vi "configuration UI.vi"() -> ()   [LabVIEW 2013, in "TDMS datalogger editor node.lvclass"]
uses:
  TDMS datalogger editor node.lvclass
  <vilib>/CEF_TreeControl/Node/NodeRef.ctl
  <vilib>/CEF_TreeControl/Node/NISE_CEF_Node.lvclass
  <vilib>/NI/AMC/Message Queue.ctl
  <vilib>/NI/AMC/Message.ctl
  <vilib>/NI/Tools/Keyed Array/KeyedArray.ctl
  <vilib>/CEF_TreeControl/Node/UserEventRef.ctl
  <vilib>/CEF_TreeControl/Controls/EventCluster.ctl
  <vilib>/NI/TBM Modules/TDMS Datalogger/module/configuration/TDMS datalogger configuration.lvclass
  <vilib>/NI/Tag Bus Data Framework/Configuration Editor/Classes/Engine Parent/Engine Parent Editor Node.lvclass
  <vilib>/NI/Tag Bus/tag/tag descriptor.lvclass
  <vilib>/NI/Tag Bus/tag/Data Type.ctl
  <vilib>/NI/Module Execution Interface/Engine Configuration/engine configuration.lvclass
  <vilib>/NI/Tag Bus/tag/tag descriptor.lvclass/tag descriptor.ctl
  <vilib>/NI/Tag Bus Module Framework/root configuration/TBM configuration.lvclass/TBM configuration.ctl
  <vilib>/NI/TBM Modules/TDMS Datalogger/module/configuration/TDMS datalogger configuration.lvclass/TDMS datalogger configuration.ctl
  TDMS datalogger editor node.lvclass/TDMS datalogger editor node.ctl
  <vilib>/NI/Tag Bus/tag/write tag name.vi
  <vilib>/NI/Tag Bus/tag/write data type.vi
  <vilib>/NI/TBM Modules/TDMS Datalogger/module/configuration/Write scans per write.vi
  <vilib>/NI/TBM Modules/TDMS Datalogger/module/configuration/Write queue size.vi
  <vilib>/NI/TBM Modules/TDMS Datalogger/module/configuration/Write Path.vi
  <vilib>/NI/TBM Modules/TDMS Datalogger/module/configuration/Write backup directory.vi
  <vilib>/NI/TBM Modules/TDMS Datalogger/module/configuration/Write channel pattern matches.vi
  <vilib>/NI/Tag Bus Module Framework/root configuration/Read instance name.vi
  <vilib>/NI/TBM Modules/TDMS Datalogger/module/configuration/Read backup directory.vi
  <vilib>/NI/TBM Modules/TDMS Datalogger/module/configuration/Read Path.vi
  <vilib>/NI/TBM Modules/TDMS Datalogger/module/configuration/Read queue size.vi
  <vilib>/NI/TBM Modules/TDMS Datalogger/module/configuration/Read scans per write.vi
  <vilib>/NI/TBM Modules/TDMS Datalogger/module/configuration/Read add enable channel.vi
  <vilib>/NI/TBM Modules/TDMS Datalogger/module/configuration/Read channel pattern matches.vi
  <vilib>/NI/Tag Bus Data Framework/Configuration Editor/Classes/Module editor node/Read Module Configuration.vi
  <vilib>/NI/Tag Bus Module Framework/root configuration/create GUID.vi
  <vilib>/NI/Tag Bus Module Framework/module configuration/TBM module configuration.lvclass
  <vilib>/NI/Tag Bus Data Framework/Configuration Editor/Classes/Module editor node/module editor node.lvclass
  <vilib>/CEF_TreeControl/NISE_CEF_TreeControl.lvlib
  <vilib>/NI/Tools/Keyed Array/Tools_KeyedArray.lvlib
  <vilib>/NI/AMC/AMC.lvlib
panel:
  in  "Tab Control":T1(tab)
  in  "channels":i32(listbox)
  in  "remove":bool
  in  "avail tags":i32(listbox)=-1
  in  "add all":bool
  in  "add1":bool
  out "Enable Tag":string
  in  "history error":bool
  in  "path error":bool
  in  "Historical Directory":path
  in  "use enable channel":bool
  in  "recalc":bool
  out "Approximate memory usage":dbl
  in  "queue size":i32=2
  in  "scans per write":i32=20
  in  "File Path":path
  in  "Channel Subscription Pattern Matches":string[](array[string])
  in  "Enable Dynamic Mapping":bool
  in  "user event":T2
  in  "main queue":T3
  in  "node ref":T4
  # "kB"
  # "Note: This value ignores dynamic mapping"
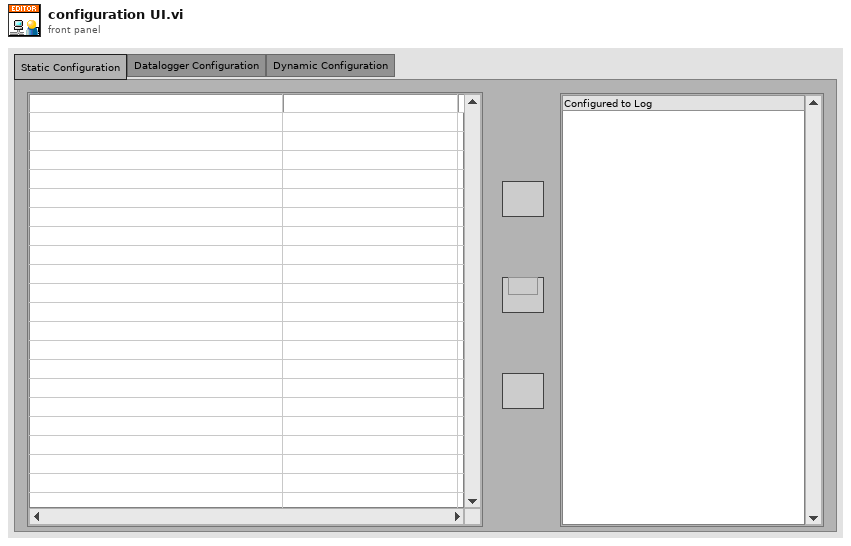
[diagram p1: front panel]
types:
  T1 = enum32{"Static Configuration", "Datalogger Configuration", "Dynamic Configuration"}
  T2 = typedef "NISE_CEF_Node.lvclass/UserEventRef.ctl" = refnum<user-event>
  T3 = typedef "AMC.lvlib/Message Queue.ctl" = refnum<queue>
  T4 = typedef "NISE_CEF_Node.lvclass/NodeRef.ctl" = refnum<data-value>
  T5 = typedef "NISE_CEF_TreeControl.lvlib/EventCluster.ctl" = cluster{"command":string, "data":string}
  T6 = typedef "tag bus.lvlib/tag descriptor.lvclass/Data Type.ctl" = enum16{"Double", "Single", "I64", "I32", "I16", "I8", "U64", "U32", "U16", "U8", "Boolean", "String", "Array of Double", "Array of Single", "Array of I64", "Array of I32", "Array of I16", "Array of I8", "Array of U64", "Array of U32", "Array of U16", "Array of U8", "Array of Boolean", "Array of String"}
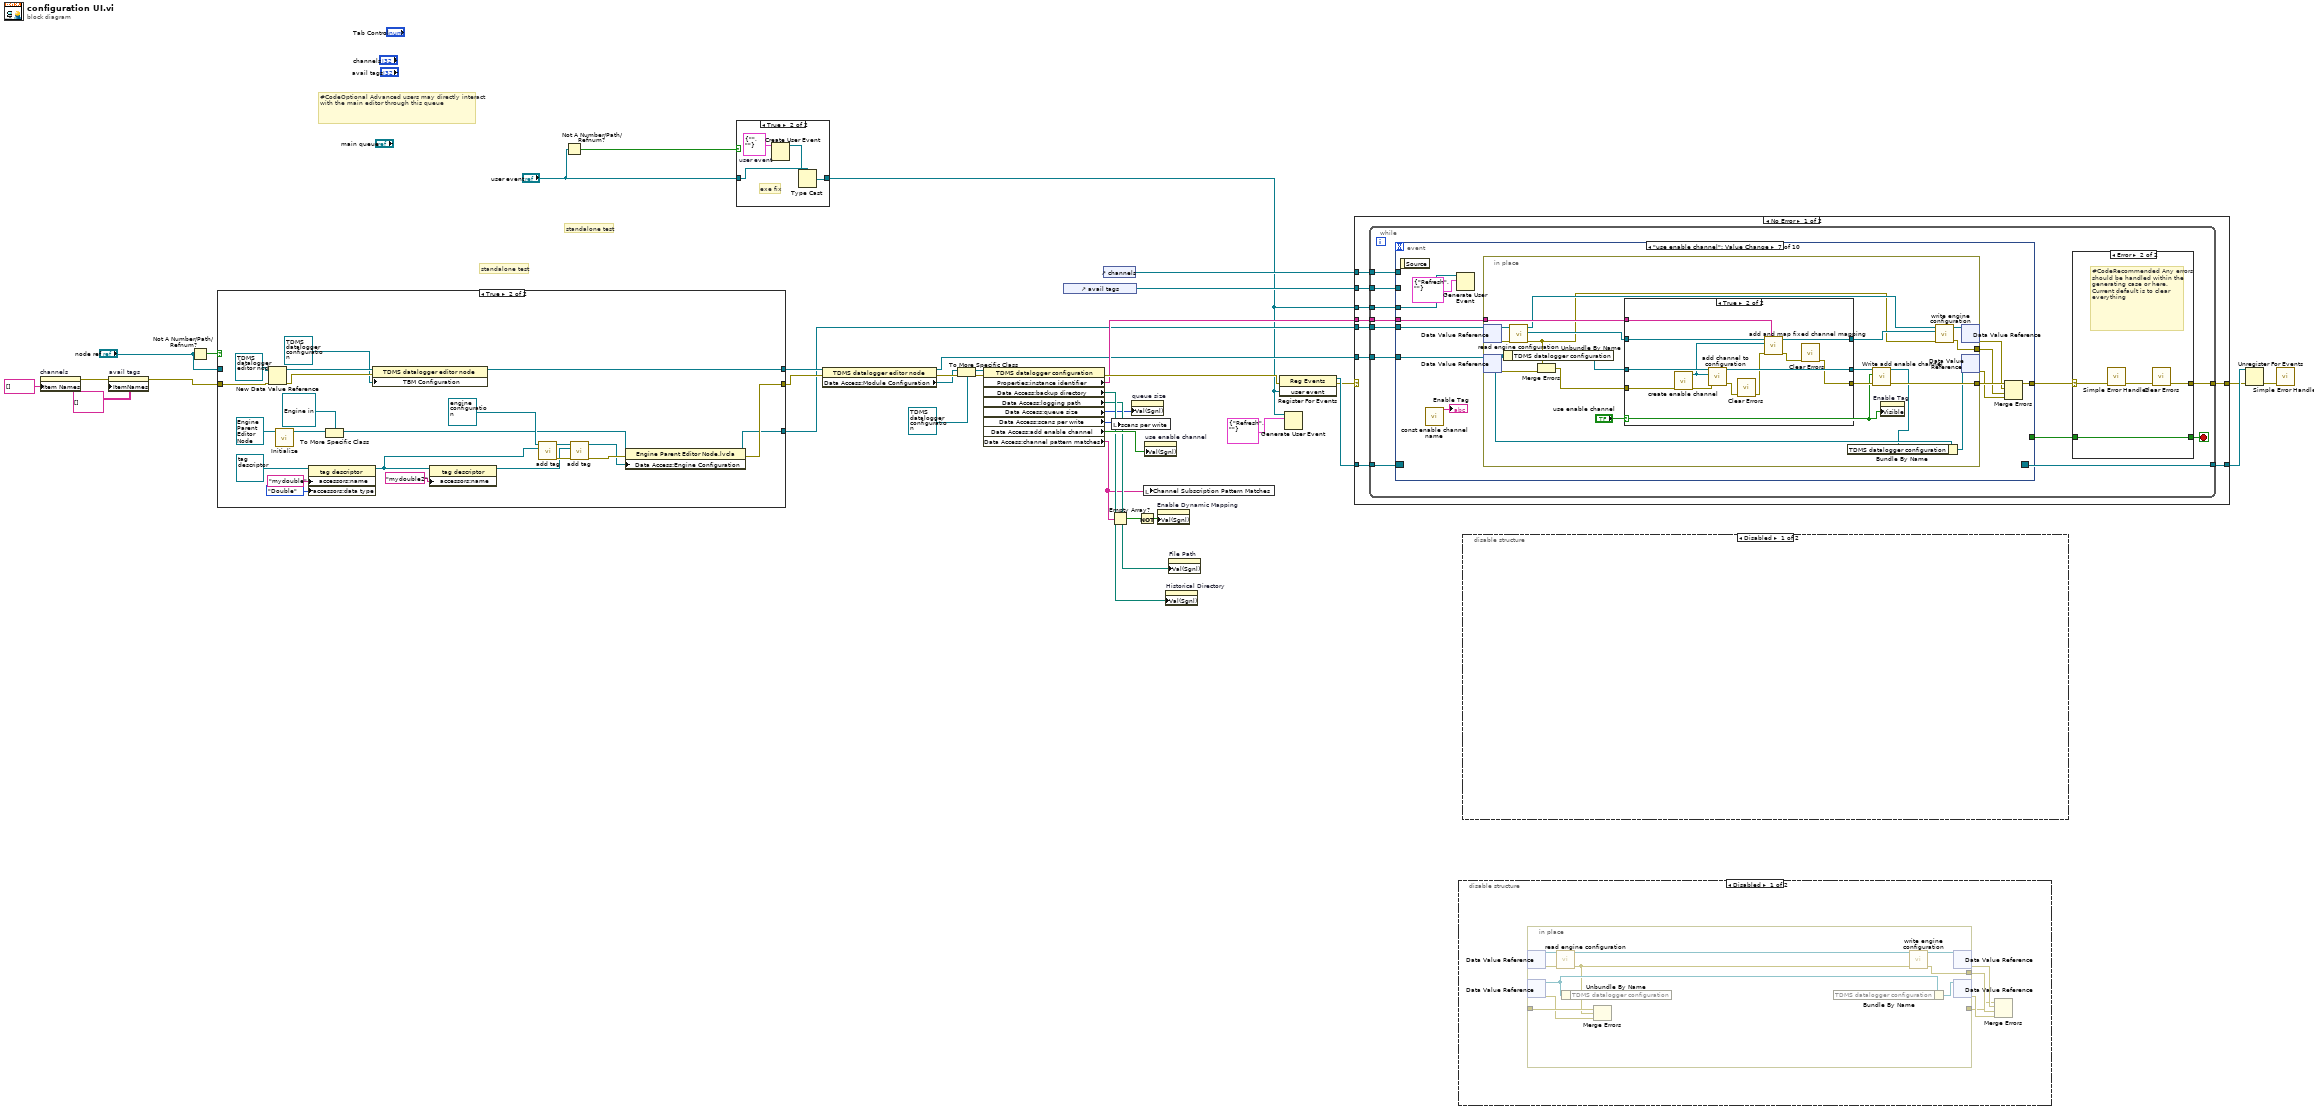
[diagram p0: block diagram]
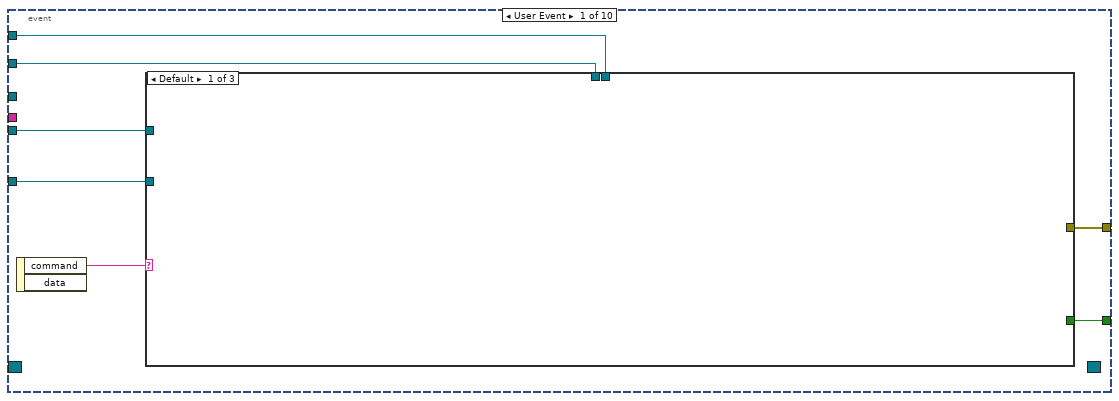
[diagram p4: hidden frame]
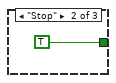
[diagram p5: hidden frame]
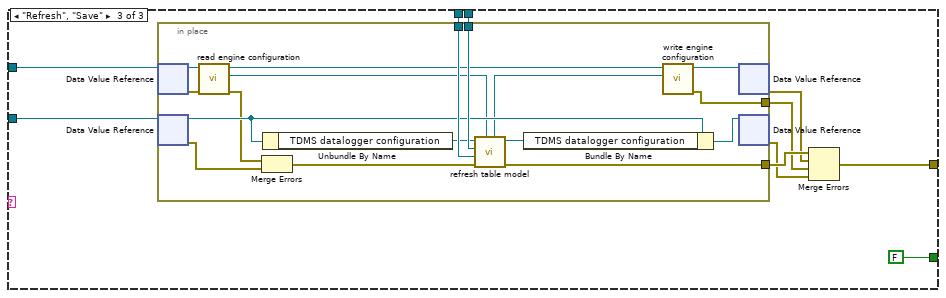
[diagram p6: hidden frame]
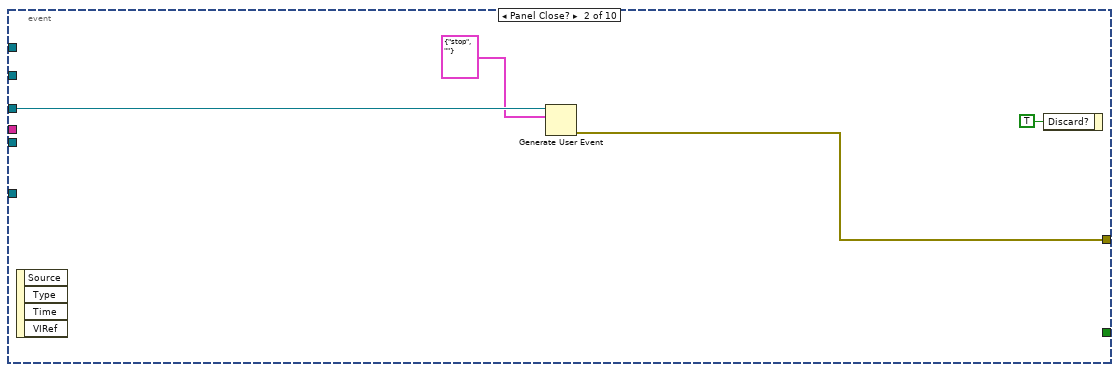
[diagram p7: hidden frame]
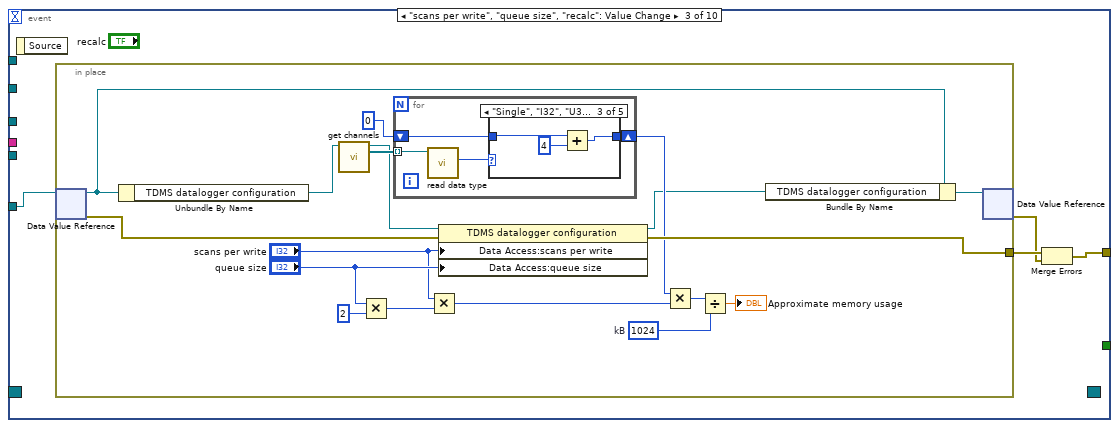
[diagram p8: hidden frame]
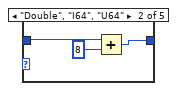
[diagram p10: hidden frame]
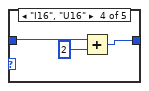
[diagram p11: hidden frame]
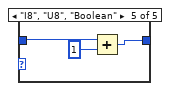
[diagram p12: hidden frame]
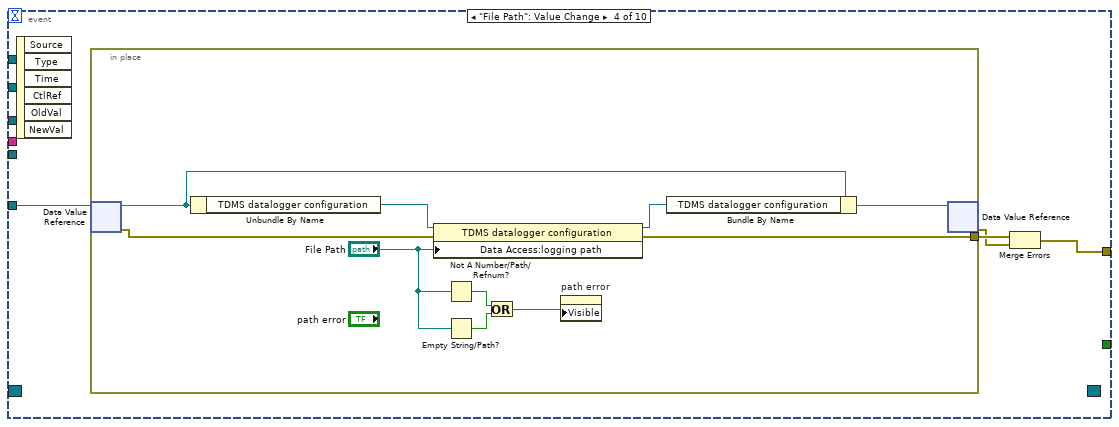
[diagram p13: hidden frame]
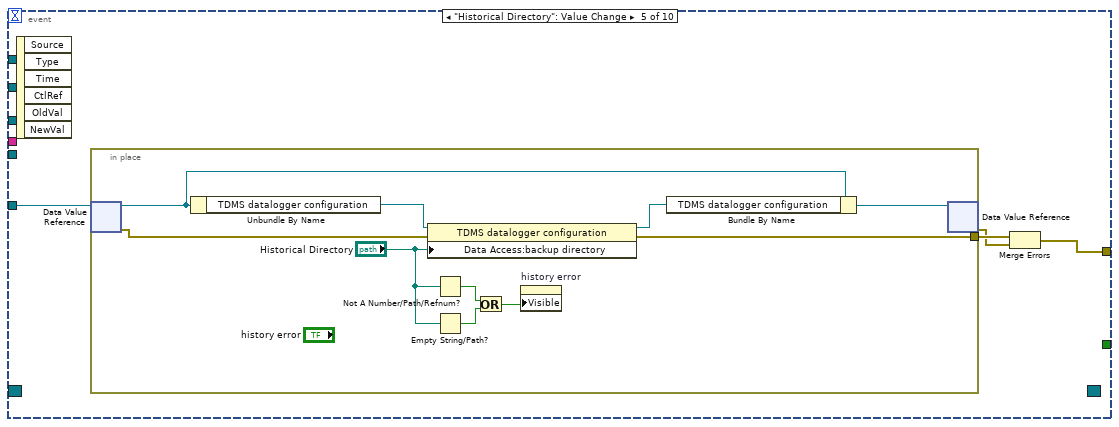
[diagram p14: hidden frame]
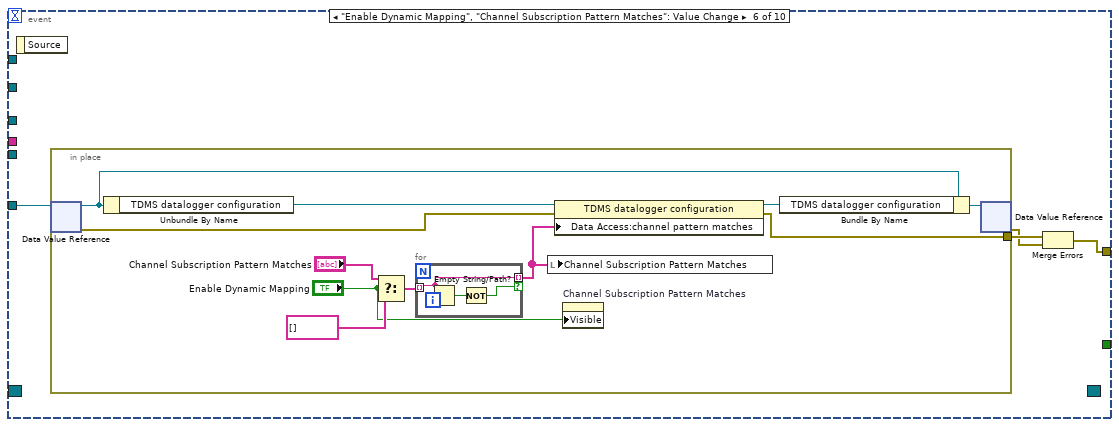
[diagram p15: hidden frame]
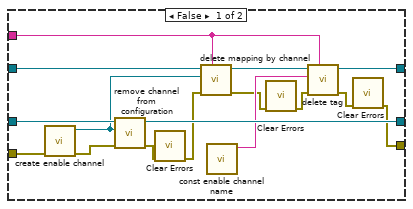
[diagram p16: hidden frame]
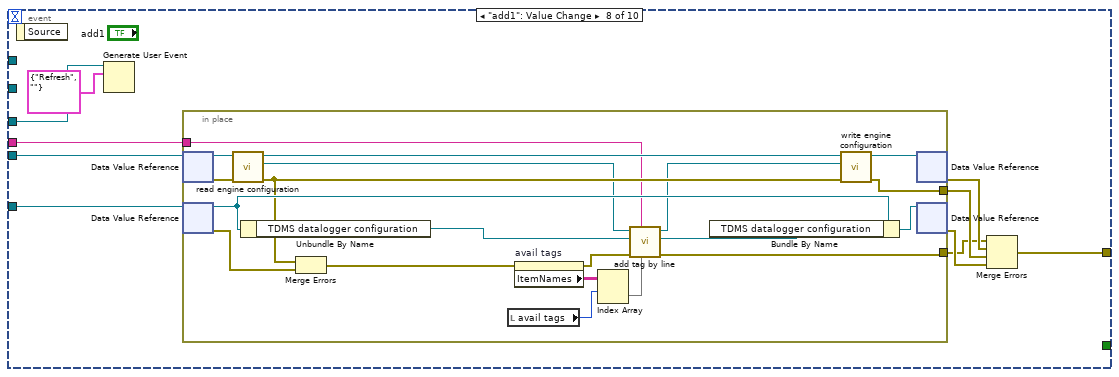
[diagram p17: hidden frame]
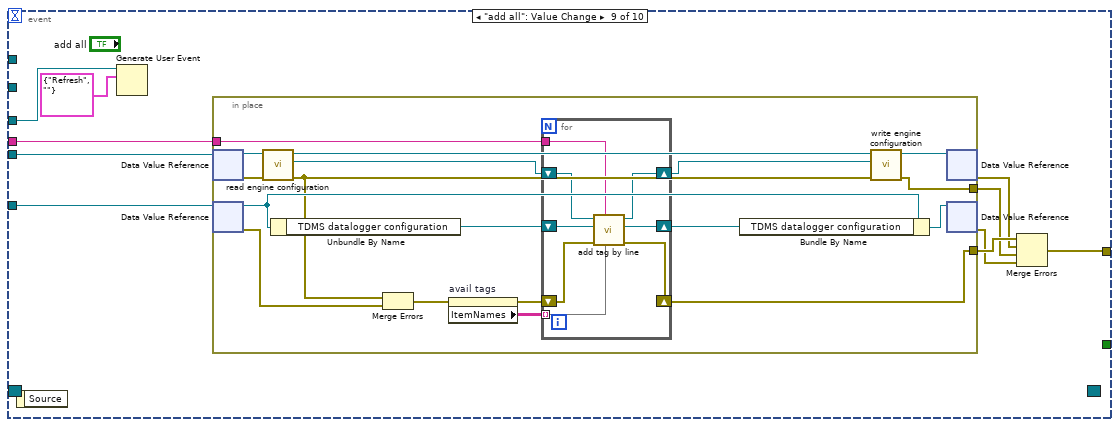
[diagram p18: hidden frame]
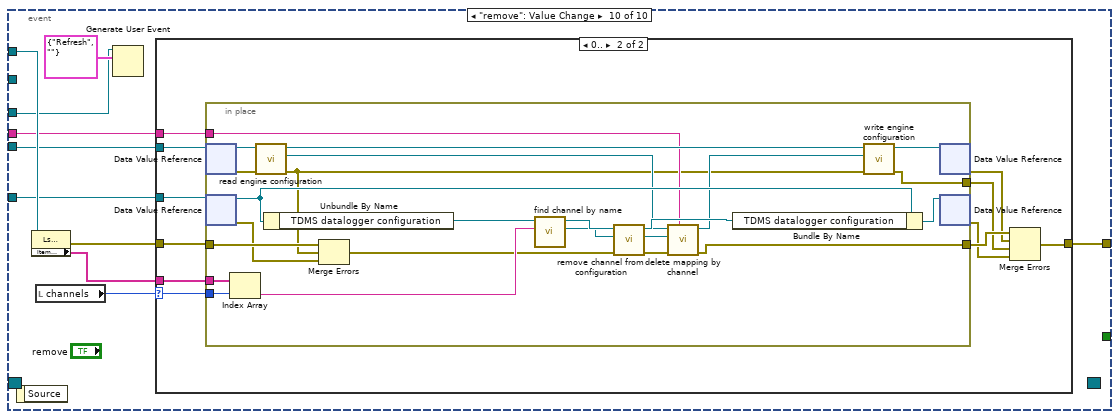
[diagram p19: hidden frame]
diagram:
  # "standalone test"
  # "standalone test"
  # "#CodeOptional Advanced users may directly interact with the main editor through this queue"
  n1 = property on="channels" class="LstBox (strict)"("Item Names"=string[] []) -> (error out=w16:errorcluster)  [unwired: 2 in, 1 out]
  n2 = property on="avail tags" class="MCListbox (strict)"(error in=w16, "ItemNames"=string[][] [] ("Item Names")) -> (error out=w5:errorcluster)  [unwired: 1 in, 1 out]
  n3 = Not A Number/Path/Refnum?(number/path/refnum="node ref") -> (NaN/Path/Refnum?=w7:bool)
  n4 = case shown="True" w7 {
    tunnel: "node ref" -> [w42 _]
    tunnel: [w41 w66] -> w9
    tunnel: [w40 w47] -> w8
    tunnel: [w39 w45] -> w4
    tunnel: w5 -> [w37 w49]
    frame False {
      n5 = call <vilib>:"locate engine.vi"("error in"=w37, "component"=w42) -> ("error out"=w38:errorcluster, "engine"=w39:refnum<data-value>)  [unwired: 8 in]
      n6 = To More Specific Class(target class=refnum<data-value> refnum ("data value reference"), reference=w42, error in=w38) -> (specific class reference=w41:refnum<data-value>, error out=w40:errorcluster)
    }
    frame True {
      n7 = New Data Value Reference(data value=refnum<class "TDMS datalogger editor node.lvclass"> refnum ("tag bus configurable plugin editor node"), error in=w49) -> (data value reference=w65:refnum<data-value>, error out=w50:errorcluster)
      n8 = call-dynamic "Initialize.vi"("Engine in"=refnum<class "Engine Parent Editor Node.lvclass"> refnum) -> ("data value reference"=w64:T4)  [unwired: 8 in, 2 out]
      n9 = property class="tag descriptor"(reference=refnum<class "tag descriptor.lvclass"> refnum ("tag descriptor"), "accessors:name"="mydouble" ("name"), "accessors:data type"=Data_Type."Double" ("data type")) -> (reference out=w53:refnum<class "tag descriptor.lvclass">)  [unwired: 1 in, 1 out]
      n10 = To More Specific Class(target class=refnum<data-value> refnum ("data value reference"), reference=w64) -> (specific class reference=w46:refnum<data-value>)  [unwired: 1 in, 1 out]
      n11 = property class="TDMS datalogger editor node"(reference=w65, error in=w50, "TBM Configuration"=refnum<class "TDMS datalogger configuration.lvclass"> refnum ("TDMS datalogger configuration")) -> (reference out=w66:refnum<data-value>)  [unwired: 1 out]
      n12 = property class="tag descriptor"(reference=w53, "accessors:name"="mydouble2" ("name")) -> (reference out=w54:refnum<class "tag descriptor.lvclass">)  [unwired: 1 in, 1 out]
      n13 = call <vilib>:"add tag.vi"("tag descriptor"=w53, "engine configuration in"=refnum<class "engine configuration.lvclass"> refnum ("Engine Configuration")) -> ("error out"=w57:errorcluster, "engine configuration out"=w56:refnum<class "engine configuration.lvclass">)  [unwired: 8 in]
      n14 = call <vilib>:"add tag.vi"("error in"=w57, "tag descriptor"=w54, "engine configuration in"=w56) -> ("error out"=w55:errorcluster, "engine configuration out"=w44:refnum<class "engine configuration.lvclass">)  [unwired: 7 in]
      n15 = property class="Engine Parent Editor Node.lvcla"(reference=w46, error in=w55, "Data Access:Engine Configuration"=w44) -> (reference out=w45:refnum<data-value>, error out=w47:errorcluster)
    }
  }
  n16 = Not A Number/Path/Refnum?(number/path/refnum="user event") -> (NaN/Path/Refnum?=w11:bool)
  n17 = case shown="True" w11 {
    tunnel: [w67 w70] -> w3
    tunnel: "user event" -> [w67 w71]
    frame False {
    }
    frame True {
      w68 = T5 {"command"="", "data"=""}  # user event
      # "exe fix"
      n18 = Create User Event(user event datatype=w68) -> (user event=w69:refnum<user-event>)  [unwired: 1 in, 1 out]
      n19 = Type Cast(type=w71, x=w69) -> (*(type *) &x=w70:T2)
    }
  }
  n20 = property class="TDMS datalogger editor node"(reference=w9, error in=w8) -> (reference out=w12:refnum<data-value>, error out=w33:errorcluster, "Data Access:Module Configuration"=w23:refnum<class "TBM module configuration.lvclass">)
  n21 = To More Specific Class(target class=refnum<class "TDMS datalogger configuration.lvclass"> refnum ("TDMS datalogger configuration"), reference=w23, error in=w33) -> (specific class reference=w21:refnum<class "TDMS datalogger configuration.lvclass">, error out=w24:errorcluster)
  n22 = property class="TDMS datalogger configuration"(reference=w21, error in=w24) -> (error out=w20:errorcluster, "Properties:instance identifier"=w17:string, "Data Access:backup directory"=w30:path, "Data Access:logging path"=w29:path, "Data Access:queue size"=w28:i32, "Data Access:scans per write"=w32:i32, "Data Access:add enable channel"=w31:bool, "Data Access:channel pattern matches"=w27:string[])  [unwired: 1 out]
  n23 = control-ref of="avail tags"() -> (w18:refnum<vi>)
  n24 = control-ref of="channels"() -> (w19:refnum<vi>)
  n25 = Empty Array?(array=w27) -> (empty?=w25:bool)
  n26 = local write "scans per write"(w32) -> ()
  n27 = property on="queue size" class="DigNum (strict)"("Val(Sgnl)"=w28) -> ()  [unwired: 2 in, 2 out]
  n28 = Not(x=w25) -> (.not. x?=w26:bool)
  n29 = local write "Channel Subscription Pattern Matches"(w27) -> ()
  n30 = property on="use enable channel" class="Bool (strict)"("Val(Sgnl)"=w31) -> ()  [unwired: 2 in, 2 out]
  n31 = property on="Enable Dynamic Mapping" class="Bool (strict)"("Val(Sgnl)"=w26) -> ()  [unwired: 2 in, 2 out]
  n32 = property on="Historical Directory" class="Path"("Val(Sgnl)"=w30) -> ()  [unwired: 2 in, 2 out]
  n33 = property on="File Path" class="Path"("Val(Sgnl)"=w29) -> ()  [unwired: 2 in, 2 out]
  n34 = register-events(error in=w20, w3) -> (reference out=w36:refnum<event-registration>, error out=w1:errorcluster)  [unwired: 1 in]
  n35 = Generate User Event(user event=w3, event data cluster=T5 {"command"="Refresh", "data"=""} ("event data")) -> ()  [unwired: 2 in, 2 out]
  n36 = case shown="No Error" w1 {
    selector: w1 -> [_ w393]
    tunnel: w36 -> [w80 w392]
    tunnel: [w79 w392] -> w35
    tunnel: w19 -> [w78 _]
    tunnel: w18 -> [w77 _]
    tunnel: w17 -> [w76 _]
    tunnel: [w75 w393] -> w13
    tunnel: w12 -> [w74 _]
    tunnel: w4 -> [w73 _]
    tunnel: w3 -> [w72 _]
    frame No Error {
      n37 = while {
        tunnel: w80 -> [w92]
        tunnel: [w91] -> w79
        tunnel: w78 -> [w87]
        tunnel: w77 -> [w86]
        tunnel: w76 -> [w81]
        tunnel: w73 -> [w85]
        tunnel: w74 -> [w84]
        tunnel: w72 -> [w83]
        tunnel: [w88] -> w75
        stop <- w89 stop-if-true
        n38 = event shown="[6] \"use enable channel\": Value Change" {
          selector: w92 -> [_ _ _ _ _ _ _ _ _ _]
          dyn-events: [_ _ _ _ _ _ _ _ _ _] -> w91
          timeout: _ -> [_ _ _ _ _ _ _ _ _ _]
          tunnel: [w105 _ _ _ _ _ _ _ _ _] -> w82
          tunnel: [w103 w136 w139 w179 w193 w205 w229 w282 w314 w356] -> w90
          tunnel: w87 -> [w100 _ _ _ _ _ _ _ _ w354]
          tunnel: w86 -> [w99 _ _ _ _ _ _ _ _ _]
          tunnel: w85 -> [w102 _ _ _ _ _ w227 w283 w312 w347]
          tunnel: w84 -> [w101 _ w140 w178 w192 w206 w228 w284 w313 w348]
          tunnel: w83 -> [_ w135 _ _ _ _ w231 w289 w319 w349]
          tunnel: w81 -> [_ _ _ _ _ _ w233 w281 w311 w352]
          event User Event {
            n39 = event-data() -> ("command"=w104:string)  [unwired: 1 in, 1 out]
            n40 = case shown="Default" w104 {
              tunnel: [_ TRUE FALSE] -> w105
              tunnel: [_ _ w112] -> w103
              tunnel: w102 -> [_ _ w111]
              tunnel: w101 -> [_ _ w110]
              tunnel: w100 -> [_ _ w114]
              tunnel: w99 -> [_ _ w113]
              frame Default {
              }
              frame "Stop" {
              }
              frame "Refresh", "Save" {
                n41 = in-place {
                  in-place-border: [w133] -> w115
                  in-place-border: w114 -> [w132]
                  in-place-border: w113 -> [w131]
                  in-place-border: [w117] -> w109
                  n42 = in-place-dvr #1(w111) -> (w121:refnum<class "Engine Parent Editor Node.lvclass">, w122:errorcluster)
                  n43 = in-place-dvr #2(w110) -> (w128:refnum<class "TDMS datalogger editor node.lvclass">, w125:errorcluster)
                  n44 = call <vilib>:"read engine configuration.vi"("error in"=w122, "Engine Parent Editor Node in"=w121) -> ("error out"=w118:errorcluster, "engine configuration"=w119:refnum<class "engine configuration.lvclass">, "Engine Parent Editor Node out"=w120:refnum<class "Engine Parent Editor Node.lvclass">)  [unwired: 7 in]
                  n45 = Merge Errors(w118, w125) -> (w130:errorcluster)
                  n46 = Unbundle By Name(w128) -> ("TDMS datalogger configuration"=w129:refnum<class "TDMS datalogger configuration.lvclass">)
                  n47 = call "refresh table model.vi"("engine configuration"=w119, "error in"=w130, "avail tags"=w131, "chan table"=w132, "TDMS datalogger configuration"=w129) -> ("error out"=w133:errorcluster, "TDMS datalogger configuration out"=w126:refnum<class "TDMS datalogger configuration.lvclass">, "engine configuration out"=w123:refnum<class "engine configuration.lvclass">)  [unwired: 4 in]
                  n48 = Bundle By Name(cluster=w128, "TDMS datalogger configuration"=w126) -> (w127:refnum<class "TDMS datalogger editor node.lvclass">)
                  n49 = call <vilib>:"write engine configuration.vi"("engine configuration"=w123, "Engine Parent Editor Node in"=w120) -> ("error out"=w117:errorcluster, "Engine Parent Editor Node out"=w124:refnum<class "Engine Parent Editor Node.lvclass">)  [unwired: 8 in]
                  n50 = in-place-dvr #1(w124) -> (w108:errorcluster)  [unwired: 1 out]
                  n51 = in-place-dvr #2(w127) -> (w107:errorcluster)  [unwired: 1 out]
                }
                n52 = Merge Errors(w115, w108, w109, w107) -> (w112:errorcluster)
              }
            }
          }
          event Panel Close? {
            n53 = event-data() -> ()  [unwired: 1 in, 4 out]
            n54 = Generate User Event(user event=w135, event data cluster=T5 {"command"="stop", "data"=""} ("event data")) -> (error out=w136:errorcluster)  [unwired: 2 in, 1 out]
            n55 = event-data("Discard?"=TRUE) -> ()  [unwired: 1 in, 1 out]
          }
          event "scans per write", "queue size", "recalc": Value Change {
            n56 = event-data() -> ()  [unwired: 1 in, 1 out]
            n57 = in-place {
              in-place-border: [w159] -> w141
              w153 = u32 1024  # kB
              n58 = in-place-dvr #3(w140) -> (w145:refnum<class "TDMS datalogger editor node.lvclass">, w146:errorcluster)
              n59 = Unbundle By Name(w145) -> ("TDMS datalogger configuration"=w143:refnum<class "TDMS datalogger configuration.lvclass">)
              n60 = call-dynamic "get channels.vi"("module configuration in"=w143) -> ("channels"=w149:refnum<class "TBM channel.lvclass">[], "module configuration out"=w147:refnum<class "TDMS datalogger configuration.lvclass">)  [unwired: 9 in]
              n61 = Multiply(x="queue size", y=2 ("x")) -> (x*y=w158:i32)
              n62 = for {
                shift-right: [w162] -> w150
                shift-left: u32 0 -> [w163]
                tunnel: w149 -> [w160] mode=indexing
                n63 = call <vilib>:"read data type.vi"("system tag in"=w160) -> ("data type"=w161:T6)  [unwired: 8 in, 2 out]
                n64 = case shown="\"Single\", \"I32\", \"U32\"" w161 {
                  tunnel: w163 -> [w164 w167 w170 w173 w176]
                  tunnel: [w164 w166 w169 w172 w175] -> w162
                  frame Default {
                  }
                  frame "Double", "I64", "U64" {
                    n65 = Add(x=w167, y=u32 8) -> (x+y=w166:u32)
                  }
                  frame "Single", "I32", "U32" {
                    n66 = Add(x=w170, y=u32 4) -> (x+y=w169:u32)
                  }
                  frame "I16", "U16" {
                    n67 = Add(x=w173, y=u32 2) -> (x+y=w172:u32)
                  }
                  frame "I8", "U8", "Boolean" {
                    n68 = Add(x=w176, y=u32 1) -> (x+y=w175:u32)
                  }
                }
              }
              n69 = Multiply(x="scans per write", y=w158) -> (x*y=w152:i32)
              n70 = property class="TDMS datalogger configuration"(reference=w147, error in=w146, "Data Access:scans per write"="scans per write", "Data Access:queue size"="queue size") -> (reference out=w142:refnum<class "TDMS datalogger configuration.lvclass">, error out=w159:errorcluster)
              n71 = Multiply(x=w150, y=w152) -> (x*y=w154:u32)
              n72 = Divide(x=w154, y=w153) -> (x/y=→"Approximate memory usage":dbl)
              n73 = Bundle By Name(cluster=w145, "TDMS datalogger configuration"=w142) -> (w144:refnum<class "TDMS datalogger editor node.lvclass">)
              n74 = in-place-dvr #3(w144) -> (w138:errorcluster)  [unwired: 1 out]
            }
            n75 = Merge Errors(w141, w138) -> (w139:errorcluster)
          }
          event "File Path": Value Change {
            n76 = event-data() -> ()  [unwired: 1 in, 6 out]
            n77 = in-place {
              in-place-border: [w190] -> w180
              n78 = in-place-dvr #4(w178) -> (w181:refnum<class "TDMS datalogger editor node.lvclass">, w184:errorcluster)
              n79 = Unbundle By Name(w181) -> ("TDMS datalogger configuration"=w185:refnum<class "TDMS datalogger configuration.lvclass">)
              n80 = property class="TDMS datalogger configuration"(reference=w185, error in=w184, "Data Access:logging path"="File Path") -> (reference out=w183:refnum<class "TDMS datalogger configuration.lvclass">, error out=w190:errorcluster)
              n81 = Not A Number/Path/Refnum?(number/path/refnum="File Path") -> (NaN/Path/Refnum?=w187:bool)
              n82 = Empty String/Path?(string/path="File Path") -> (empty?=w188:bool)
              n83 = Or(x=w187, y=w188) -> (x .or. y?=w186:bool)
              n84 = property on="path error" class="Bool"("Visible"=w186) -> ()  [unwired: 2 in, 2 out]
              n85 = Bundle By Name(cluster=w181, "TDMS datalogger configuration"=w183) -> (w182:refnum<class "TDMS datalogger editor node.lvclass">)
              n86 = in-place-dvr #4(w182) -> (w177:errorcluster)  [unwired: 1 out]
            }
            n87 = Merge Errors(w180, w177) -> (w179:errorcluster)
          }
          event "Historical Directory": Value Change {
            n88 = event-data() -> ()  [unwired: 1 in, 6 out]
            n89 = in-place {
              in-place-border: [w198] -> w194
              n90 = in-place-dvr #5(w192) -> (w203:refnum<class "TDMS datalogger editor node.lvclass">, w195:errorcluster)
              n91 = Unbundle By Name(w203) -> ("TDMS datalogger configuration"=w196:refnum<class "TDMS datalogger configuration.lvclass">)
              n92 = property class="TDMS datalogger configuration"(reference=w196, error in=w195, "Data Access:backup directory"="Historical Directory") -> (reference out=w197:refnum<class "TDMS datalogger configuration.lvclass">, error out=w198:errorcluster)
              n93 = Not A Number/Path/Refnum?(number/path/refnum="Historical Directory") -> (NaN/Path/Refnum?=w201:bool)
              n94 = Empty String/Path?(string/path="Historical Directory") -> (empty?=w202:bool)
              n95 = Or(x=w201, y=w202) -> (x .or. y?=w199:bool)
              n96 = property on="history error" class="Bool"("Visible"=w199) -> ()  [unwired: 2 in, 2 out]
              n97 = Bundle By Name(cluster=w203, "TDMS datalogger configuration"=w197) -> (w204:refnum<class "TDMS datalogger editor node.lvclass">)
              n98 = in-place-dvr #5(w204) -> (w191:errorcluster)  [unwired: 1 out]
            }
            n99 = Merge Errors(w194, w191) -> (w193:errorcluster)
          }
          event "Enable Dynamic Mapping", "Channel Subscription Pattern Matches": Value Change {
            n100 = event-data() -> ()  [unwired: 1 in, 1 out]
            n101 = in-place {
              in-place-border: [w209] -> w208
              n102 = in-place-dvr #6(w206) -> (w218:refnum<class "TDMS datalogger editor node.lvclass">, w210:errorcluster)
              n103 = Unbundle By Name(w218) -> ("TDMS datalogger configuration"=w211:refnum<class "TDMS datalogger configuration.lvclass">)
              n104 = Select(t="Channel Subscription Pattern Matches", s="Enable Dynamic Mapping", f=string[] []) -> (s? t:f=w214:string[])
              n105 = for {
                tunnel: w214 -> [w222] mode=indexing
                tunnel: [w222] -> w213 mode=indexing if=w220
                n106 = Empty String/Path?(string/path=w222) -> (empty?=w221:bool)
                n107 = Not(x=w221) -> (.not. x?=w220:bool)
              }
              n108 = local write "Channel Subscription Pattern Matches"(w213) -> ()
              n109 = property class="TDMS datalogger configuration"(reference=w211, error in=w210, "Data Access:channel pattern matches"=w213) -> (reference out=w212:refnum<class "TDMS datalogger configuration.lvclass">, error out=w209:errorcluster)
              n110 = property on="Channel Subscription Pattern Matches" class="Arr (strict)"("Visible"="Enable Dynamic Mapping") -> ()  [unwired: 2 in, 2 out]
              n111 = Bundle By Name(cluster=w218, "TDMS datalogger configuration"=w212) -> (w219:refnum<class "TDMS datalogger editor node.lvclass">)
              n112 = in-place-dvr #6(w219) -> (w207:errorcluster)  [unwired: 1 out]
            }
            n113 = Merge Errors(w208, w207) -> (w205:errorcluster)
          }
          event "use enable channel": Value Change {
            n114 = event-data() -> ()  [unwired: 1 in, 1 out]
            n115 = call <vilib>:"const enable channel name.vi"() -> ("enable channel"=→"Enable Tag":string)  [unwired: 11 in]
            n116 = Generate User Event(user event=w231, event data cluster=T5 {"command"="Refresh", "data"=""} ("event data")) -> ()  [unwired: 2 in, 2 out]
            n117 = in-place {
              in-place-border: w233 -> [w252]
              in-place-border: [w249] -> w230
              in-place-border: [w243] -> w225
              n118 = in-place-dvr #7(w227) -> (w247:refnum<class "Engine Parent Editor Node.lvclass">, w245:errorcluster)
              n119 = in-place-dvr #8(w228) -> (w241:refnum<class "TDMS datalogger editor node.lvclass">, w244:errorcluster)
              n120 = Unbundle By Name(w241) -> ("TDMS datalogger configuration"=w242:refnum<class "TDMS datalogger configuration.lvclass">)
              n121 = call <vilib>:"read engine configuration.vi"("error in"=w245, "Engine Parent Editor Node in"=w247) -> ("error out"=w235:errorcluster, "engine configuration"=w246:refnum<class "engine configuration.lvclass">, "Engine Parent Editor Node out"=w237:refnum<class "Engine Parent Editor Node.lvclass">)  [unwired: 7 in]
              n122 = Merge Errors(w235, w244) -> (w234:errorcluster)
              n123 = case shown="True" "use enable channel" {
                tunnel: w252 -> [w261 w279]
                tunnel: [w262 w280] -> w236
                tunnel: w246 -> [w265 w274]
                tunnel: [w267 w278] -> w251
                tunnel: w242 -> [w268 w277]
                tunnel: [w256 w272] -> w250
                tunnel: w234 -> [w253 w269]
                frame False {
                  n124 = call <vilib>:"create enable channel.vi"("error in"=w253) -> ("error out"=w266:errorcluster, "enable channel"=w264:refnum<class "TBM channel.lvclass">)  [unwired: 9 in]
                  n125 = call <vilib>:"remove channel from configuration.vi"("error in"=w266, "TBM channel in"=w264, "TDMS datalogger configuration in"=w268) -> ("error out"=w255:errorcluster, "TDMS datalogger configuration out"=w267:refnum<class "TDMS datalogger configuration.lvclass">)  [unwired: 7 in]
                  n126 = call <vilib>:"Clear Errors.vi"("error in (no error)"=w255) -> ("error out"=w254:errorcluster)  [unwired: 6 in]
                  n127 = call <vilib>:"delete mapping by channel.vi"("owner ID"=w261, "error in"=w254, "channel"=w264, "engine configuration in"=w265) -> ("error out"=w258:errorcluster, "engine configuration out"=w263:refnum<class "engine configuration.lvclass">)  [unwired: 6 in]
                  n128 = call <vilib>:"const enable channel name.vi"() -> ("enable channel"=w260:string)  [unwired: 11 in]
                  n129 = call <vilib>:"Clear Errors.vi"("error in (no error)"=w258) -> ("error out"=w259:errorcluster)  [unwired: 6 in]
                  n130 = call <vilib>:"delete tag.vi"("owner ID"=w261, "error in"=w259, "tag name"=w260, "engine configuration in"=w263) -> ("error out"=w257:errorcluster, "engine configuration out"=w262:refnum<class "engine configuration.lvclass">)  [unwired: 6 in]
                  n131 = call <vilib>:"Clear Errors.vi"("error in (no error)"=w257) -> ("error out"=w256:errorcluster)  [unwired: 6 in]
                }
                frame True {
                  n132 = call <vilib>:"create enable channel.vi"("error in"=w269) -> ("error out"=w276:errorcluster, "enable channel"=w275:refnum<class "TBM channel.lvclass">)  [unwired: 9 in]
                  n133 = call <vilib>:"add channel to configuration.vi"("error in"=w276, "TBM channel in"=w275, "TDMS datalogger configuration in"=w277) -> ("error out"=w271:errorcluster, "TDMS datalogger configuration out"=w278:refnum<class "TDMS datalogger configuration.lvclass">)  [unwired: 7 in]
                  n134 = call <vilib>:"Clear Errors.vi"("error in (no error)"=w271) -> ("error out"=w270:errorcluster)  [unwired: 6 in]
                  n135 = call <vilib>:"add and map fixed channel mapping.vi"("module instance"=w279, "error in"=w270, "fixed channel"=w275, "engine configuration in"=w274) -> ("error out"=w273:errorcluster, "engine configuration out"=w280:refnum<class "engine configuration.lvclass">)  [unwired: 6 in]
                  n136 = call <vilib>:"Clear Errors.vi"("error in (no error)"=w273) -> ("error out"=w272:errorcluster)  [unwired: 6 in]
                }
              }
              n137 = call <vilib>:"Write add enable channel.vi"("error in (no error)"=w250, "add enable channel"="use enable channel", "TDMS datalogger configuration in"=w251) -> ("error out"=w249:errorcluster, "TDMS datalogger configuration out"=w240:refnum<class "TDMS datalogger configuration.lvclass">)  [unwired: 7 in]
              n138 = Bundle By Name(cluster=w241, "TDMS datalogger configuration"=w240) -> (w239:refnum<class "TDMS datalogger editor node.lvclass">)
              n139 = property on="Enable Tag" class="Str"("Visible"="use enable channel") -> ()  [unwired: 2 in, 2 out]
              n140 = call <vilib>:"write engine configuration.vi"("error in"=w235, "engine configuration"=w236, "Engine Parent Editor Node in"=w237) -> ("error out"=w243:errorcluster, "Engine Parent Editor Node out"=w238:refnum<class "Engine Parent Editor Node.lvclass">)  [unwired: 7 in]
              n141 = in-place-dvr #7(w238) -> (w226:errorcluster)  [unwired: 1 out]
              n142 = in-place-dvr #8(w239) -> (w224:errorcluster)  [unwired: 1 out]
            }
            n143 = Merge Errors(w230, w226, w225, w224) -> (w229:errorcluster)
          }
          event "add1": Value Change {
            n144 = event-data() -> ()  [unwired: 1 in, 1 out]
            n145 = Generate User Event(user event=w289, event data cluster=T5 {"command"="Refresh", "data"=""} ("event data")) -> ()  [unwired: 2 in, 2 out]
            n146 = in-place {
              in-place-border: [w295] -> w285
              in-place-border: [w304] -> w286
              in-place-border: w281 -> [w291]
              n147 = in-place-dvr #9(w283) -> (w306:refnum<class "Engine Parent Editor Node.lvclass">, w307:errorcluster)
              n148 = in-place-dvr #10(w284) -> (w303:refnum<class "TDMS datalogger editor node.lvclass">, w309:errorcluster)
              n149 = call <vilib>:"read engine configuration.vi"("error in"=w307, "Engine Parent Editor Node in"=w306) -> ("error out"=w302:errorcluster, "engine configuration"=w293:refnum<class "engine configuration.lvclass">, "Engine Parent Editor Node out"=w305:refnum<class "Engine Parent Editor Node.lvclass">)  [unwired: 7 in]
              n150 = Unbundle By Name(w303) -> ("TDMS datalogger configuration"=w297:refnum<class "TDMS datalogger configuration.lvclass">)
              n151 = Merge Errors(w302, w309) -> (w292:errorcluster)
              n152 = local read "avail tags"() -> (w299:i32)
              n153 = property on="avail tags" class="MCListbox (strict)"(error in=w292) -> (error out=w300:errorcluster, "ItemNames"=w298:string[][])  [unwired: 1 in, 1 out]
              n154 = Index Array(array=w298, index (row)=w299) -> (element=w301:string[])  [unwired: 1 in]
              n155 = call "add tag by line.vi"("ItemNames"=w301, "Properties:instance identifier"=w291, "error in"=w300, "TDMS datalogger configuration in"=w297, "engine configuration in"=w293) -> ("error out"=w295:errorcluster, "TDMS datalogger configuration out"=w296:refnum<class "TDMS datalogger configuration.lvclass">, "engine configuration out"=w294:refnum<class "engine configuration.lvclass">)  [unwired: 4 in]
              n156 = Bundle By Name(cluster=w303, "TDMS datalogger configuration"=w296) -> (w310:refnum<class "TDMS datalogger editor node.lvclass">)
              n157 = call <vilib>:"write engine configuration.vi"("error in"=w302, "engine configuration"=w294, "Engine Parent Editor Node in"=w305) -> ("error out"=w304:errorcluster, "Engine Parent Editor Node out"=w308:refnum<class "Engine Parent Editor Node.lvclass">)  [unwired: 7 in]
              n158 = in-place-dvr #9(w308) -> (w287:errorcluster)  [unwired: 1 out]
              n159 = in-place-dvr #10(w310) -> (w288:errorcluster)  [unwired: 1 out]
            }
            n160 = Merge Errors(w285, w287, w286, w288) -> (w282:errorcluster)
          }
          event "add all": Value Change {
            n161 = event-data() -> ()  [unwired: 1 in, 1 out]
            n162 = Generate User Event(user event=w319, event data cluster=T5 {"command"="Refresh", "data"=""} ("event data")) -> ()  [unwired: 2 in, 2 out]
            n163 = in-place {
              in-place-border: [w323] -> w318
              in-place-border: [w332] -> w317
              in-place-border: w311 -> [w321]
              n164 = in-place-dvr #11(w312) -> (w334:refnum<class "Engine Parent Editor Node.lvclass">, w335:errorcluster)
              n165 = in-place-dvr #12(w313) -> (w331:refnum<class "TDMS datalogger editor node.lvclass">, w337:errorcluster)
              n166 = call <vilib>:"read engine configuration.vi"("error in"=w335, "Engine Parent Editor Node in"=w334) -> ("error out"=w330:errorcluster, "engine configuration"=w325:refnum<class "engine configuration.lvclass">, "Engine Parent Editor Node out"=w333:refnum<class "Engine Parent Editor Node.lvclass">)  [unwired: 7 in]
              n167 = Unbundle By Name(w331) -> ("TDMS datalogger configuration"=w326:refnum<class "TDMS datalogger configuration.lvclass">)
              n168 = Merge Errors(w330, w337) -> (w322:errorcluster)
              n169 = property on="avail tags" class="MCListbox (strict)"(error in=w322) -> (error out=w328:errorcluster, "ItemNames"=w329:string[][])  [unwired: 1 in, 1 out]
              n170 = for {
                tunnel: w329 -> [w340] mode=indexing
                shift-right: [w345] -> w323
                shift-left: w328 -> [w343]
                shift-right: [w346] -> w327
                shift-left: w326 -> [w344]
                shift-right: [w341] -> w324
                shift-left: w325 -> [w342]
                tunnel: w321 -> [w339]
                n171 = call "add tag by line.vi"("ItemNames"=w340, "Properties:instance identifier"=w339, "error in"=w343, "TDMS datalogger configuration in"=w344, "engine configuration in"=w342) -> ("error out"=w345:errorcluster, "TDMS datalogger configuration out"=w346:refnum<class "TDMS datalogger configuration.lvclass">, "engine configuration out"=w341:refnum<class "engine configuration.lvclass">)  [unwired: 4 in]
              }
              n172 = Bundle By Name(cluster=w331, "TDMS datalogger configuration"=w327) -> (w338:refnum<class "TDMS datalogger editor node.lvclass">)
              n173 = call <vilib>:"write engine configuration.vi"("error in"=w330, "engine configuration"=w324, "Engine Parent Editor Node in"=w333) -> ("error out"=w332:errorcluster, "Engine Parent Editor Node out"=w336:refnum<class "Engine Parent Editor Node.lvclass">)  [unwired: 7 in]
              n174 = in-place-dvr #11(w336) -> (w316:errorcluster)  [unwired: 1 out]
              n175 = in-place-dvr #12(w338) -> (w315:errorcluster)  [unwired: 1 out]
            }
            n176 = Merge Errors(w318, w316, w317, w315) -> (w314:errorcluster)
          }
          event "remove": Value Change {
            n177 = event-data() -> ()  [unwired: 1 in, 1 out]
            n178 = property class="LstBox (strict)"(reference=w354) -> (error out=w353:errorcluster, "Item Names"=w355:string[])  [unwired: 1 in, 1 out]
            n179 = local read "channels"() -> (w351:i32)
            n180 = Generate User Event(user event=w349, event data cluster=T5 {"command"="Refresh", "data"=""} ("event data")) -> ()  [unwired: 2 in, 2 out]
            n181 = case shown="0.." w351 {
              selector: w351 -> [_ w359]
              tunnel: [w357 w364] -> w356
              tunnel: w355 -> [_ w360]
              tunnel: w353 -> [w357 w361]
              tunnel: w352 -> [_ w358]
              tunnel: w348 -> [_ w363]
              tunnel: w347 -> [_ w362]
              frame ..-1 {
              }
              frame 0.. {
                n182 = in-place {
                  in-place-border: w361 -> [w391]
                  in-place-border: [w371] -> w368
                  in-place-border: [w384] -> w367
                  in-place-border: w360 -> [w375]
                  in-place-border: w359 -> [w374]
                  in-place-border: w358 -> [w373]
                  n183 = in-place-dvr #13(w362) -> (w386:refnum<class "Engine Parent Editor Node.lvclass">, w387:errorcluster)
                  n184 = in-place-dvr #14(w363) -> (w383:refnum<class "TDMS datalogger editor node.lvclass">, w389:errorcluster)
                  n185 = Index Array(array=w375, index=w374) -> (element=w380:string)
                  n186 = call <vilib>:"read engine configuration.vi"("error in"=w387, "Engine Parent Editor Node in"=w386) -> ("error out"=w369:errorcluster, "engine configuration"=w372:refnum<class "engine configuration.lvclass">, "Engine Parent Editor Node out"=w385:refnum<class "Engine Parent Editor Node.lvclass">)  [unwired: 7 in]
                  n187 = Unbundle By Name(w383) -> ("TDMS datalogger configuration"=w377:refnum<class "TDMS datalogger configuration.lvclass">)
                  n188 = Merge Errors(w391, w369, w389) -> (w376:errorcluster)
                  n189 = call <vilib>:"find channel by name.vi"("channel name"=w380, "TDMS datalogger configuration in"=w377) -> ("channel"=w379:refnum<class "TBM channel.lvclass">, "TDMS datalogger configuration out"=w381:refnum<class "TDMS datalogger configuration.lvclass">)  [unwired: 8 in]
                  n190 = call <vilib>:"remove channel from configuration.vi"("error in"=w376, "TBM channel in"=w379, "TDMS datalogger configuration in"=w381) -> ("error out"=w382:errorcluster, "TDMS datalogger configuration out"=w378:refnum<class "TDMS datalogger configuration.lvclass">)  [unwired: 7 in]
                  n191 = call <vilib>:"delete mapping by channel.vi"("owner ID"=w373, "error in"=w382, "channel"=w379, "engine configuration in"=w372) -> ("error out"=w371:errorcluster, "engine configuration out"=w370:refnum<class "engine configuration.lvclass">)  [unwired: 6 in]
                  n192 = Bundle By Name(cluster=w383, "TDMS datalogger configuration"=w378) -> (w390:refnum<class "TDMS datalogger editor node.lvclass">)
                  n193 = call <vilib>:"write engine configuration.vi"("error in"=w369, "engine configuration"=w370, "Engine Parent Editor Node in"=w385) -> ("error out"=w384:errorcluster, "Engine Parent Editor Node out"=w388:refnum<class "Engine Parent Editor Node.lvclass">)  [unwired: 7 in]
                  n194 = in-place-dvr #13(w388) -> (w366:errorcluster)  [unwired: 1 out]
                  n195 = in-place-dvr #14(w390) -> (w365:errorcluster)  [unwired: 1 out]
                }
                n196 = Merge Errors(w368, w366, w367, w365) -> (w364:errorcluster)
              }
            }
          }
        }
        n197 = case shown="Error" w90 {
          selector: w90 -> [w93 w97]
          tunnel: [w94 w98] -> w89
          tunnel: w82 -> [w94 w98]
          tunnel: [w93 w95] -> w88
          frame No Error {
          }
          frame Error {
            # "#CodeRecommended Any errors should be handled within the generating case or here. Current default is to clear everything"
            n198 = call <vilib>:"Simple Error Handler.vi"("error in (no error)"=w97) -> ("error out"=w96:errorcluster)  [unwired: 4 in, 4 out]
            n199 = call <vilib>:"Clear Errors.vi"("error in (no error)"=w96) -> ("error out"=w95:errorcluster)  [unwired: 6 in]
          }
        }
      }
    }
    frame Error {
    }
  }
  n200 = disable-structure shown="Disabled" {
    frame Disabled {
      n201 = in-place {
        in-place-border: _ -> [w407]
        in-place-border: [_] -> w394
        in-place-border: [w400] -> w395
        n202 = in-place-dvr #15() -> (w402:refnum<class "Engine Parent Editor Node.lvclass">, w403:errorcluster)  [unwired: 1 in]
        n203 = in-place-dvr #16() -> (w399:refnum<class "TDMS datalogger editor node.lvclass">, w405:errorcluster)  [unwired: 1 in]
        n204 = call <vilib>:"read engine configuration.vi"("error in"=w403, "Engine Parent Editor Node in"=w402) -> ("error out"=w398:errorcluster, "Engine Parent Editor Node out"=w401:refnum<class "Engine Parent Editor Node.lvclass">)  [unwired: 7 in, 1 out]
        n205 = Unbundle By Name(w399) -> ()  [unwired: 1 out]
        n206 = Merge Errors(w407, w398, w405) -> ()  [unwired: 1 out]
        n207 = Bundle By Name(cluster=w399) -> (w406:refnum<class "TDMS datalogger editor node.lvclass">)  [unwired: 1 in]
        n208 = call <vilib>:"write engine configuration.vi"("error in"=w398, "Engine Parent Editor Node in"=w401) -> ("error out"=w400:errorcluster, "Engine Parent Editor Node out"=w404:refnum<class "Engine Parent Editor Node.lvclass">)  [unwired: 8 in]
        n209 = in-place-dvr #15(w404) -> (w396:errorcluster)  [unwired: 1 out]
        n210 = in-place-dvr #16(w406) -> (w397:errorcluster)  [unwired: 1 out]
      }
      n211 = Merge Errors(w394, w396, w395, w397) -> ()  [unwired: 1 out]
    }
    frame Enabled {
    }
  }
  n212 = disable-structure shown="Disabled" {
    frame Disabled {
    }
    frame Enabled {
    }
  }
  n213 = Unregister For Events(event registration refnum=w35, error in=w13) -> (error out=w34:errorcluster)
  n214 = call <vilib>:"Simple Error Handler.vi"("error in (no error)"=w34) -> ()  [unwired: 4 in, 5 out]
